vi "XY Graph Shift Plot Arrays.vi"(6 "Rotate":bool, 8 "Error In":errorcluster, 9 "Shift [index value] (0)":dbl, 10 "Y Array":dbl[](array[numeric]), 11 "X Array":dbl[](array[numeric])) -> (0 "Error Out":errorcluster, 2 "Y Array (shifted)":dbl[](array[numeric]), 3 "X Array (out)":dbl[](array[numeric]))   [LabVIEW 2021, in "XY Graph Add-Ons.lvlib"]
uses:
  XY Graph Add-Ons.lvlib
  9bdb4e87-38b8-4919-ab0a-2a6fc2bcb965.vi
  <vilib>/Utility/error.llb/Error Cluster From Error Code.vi
  <vilib>/ErrorRing/Error Ring.xnode
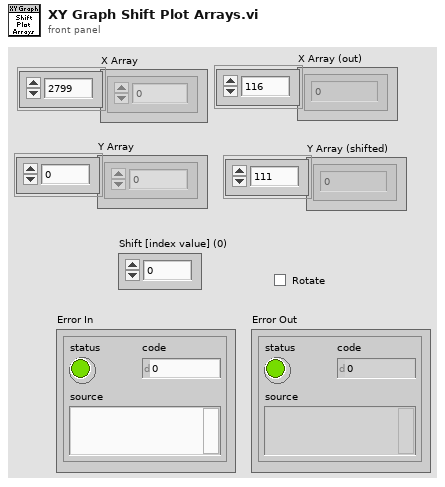
[diagram p1: front panel]
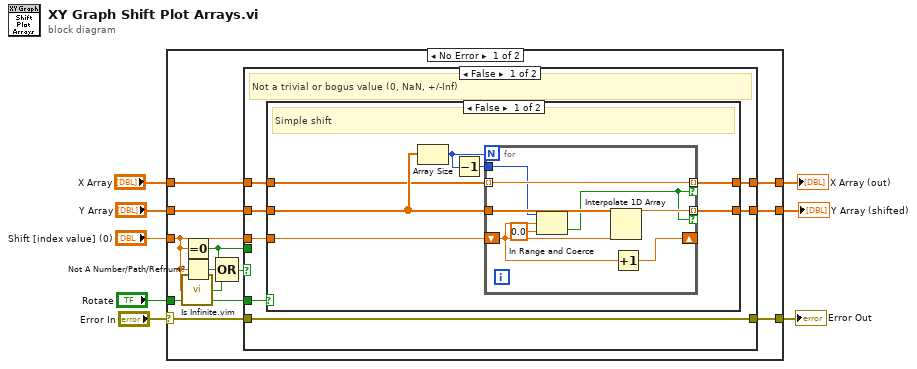
[diagram p0: block diagram]
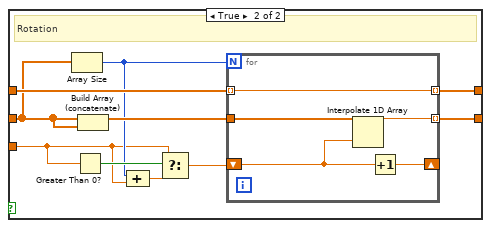
[diagram p2: hidden frame]
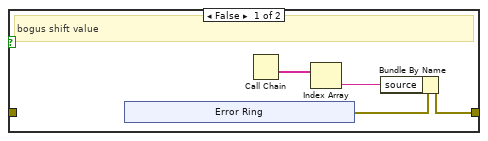
[diagram p4: hidden frame]
diagram:
  n1 = case shown="No Error" "Error In" {
    selector: "Error In" -> [w10 w72]
    tunnel: "Y Array" -> [w20 w74]
    tunnel: [w19 w74] -> w7
    tunnel: "Shift [index value] (0)" -> [w13 _]
    tunnel: "X Array" -> [w16 w73]
    tunnel: [w15 w73] -> w4
    tunnel: "Rotate" -> [w14 _]
    tunnel: [w9 w72] -> w1
    frame No Error {
      n2 = call "Is Infinite.vim"("Value"=w13) -> ("Is Infinite?"=w12:bool)
      n3 = Equal To 0?(x=w13) -> (x = 0?=w11:bool)
      n4 = Not A Number/Path/Refnum?(number/path/refnum=w13) -> (NaN/Path/Refnum?=w17:bool)
      n5 = Compound Arithmetic op=OR(w11, w17, w12) -> (w18:bool)
      n6 = case shown="False" w18 {
        tunnel: w20 -> [w27 w62]
        tunnel: [w26 w62] -> w19
        tunnel: w13 -> [w25 _]
        tunnel: w16 -> [w24 w61]
        tunnel: [w23 w61] -> w15
        tunnel: w14 -> [w22 _]
        tunnel: w11 -> [_ w60]
        tunnel: w10 -> [w21 w59]
        tunnel: [w21 w58] -> w9
        frame False {
          # "Not a trivial or bogus value (0, NaN, +/-Inf)"
          n7 = case shown="False" w22 {
            tunnel: w27 -> [w34 w49]
            tunnel: [w33 w52] -> w26
            tunnel: w25 -> [w32 w43]
            tunnel: w24 -> [w31 w51]
            tunnel: [w30 w50] -> w23
            frame False {
              # "Simple shift"
              n8 = Array Size(array=w34) -> (size(s)=w29:i32)
              n9 = Decrement(x=w29) -> (x-1=w28:i32)
              n10 = for {
                N: w29 -> [_]
                tunnel: w34 -> [w42]
                shift-right: [w40] -> _
                shift-left: w32 -> [w38]
                tunnel: [w41] -> w33 mode=indexing if=w35
                tunnel: w31 -> [w39] mode=indexing
                tunnel: [w39] -> w30 mode=indexing if=w35
                tunnel: w28 -> [w36]
                n11 = In Range and Coerce(upper limit=w36, x=w38, lower limit=0.0) -> (In Range?=w35:bool)  [unwired: 1 out]
                n12 = Interpolate 1D Array(1:w38, 2:w42) -> (0:w41:dbl)
                n13 = Increment(x=w38) -> (x+1=w40:dbl)
              }
            }
            frame True {
              # "Rotation"
              n14 = Array Size(array=w49) -> (size(s)=w46:i32)
              n15 = Greater Than 0?(x=w43) -> (x > 0?=w47:bool)
              n16 = Build Array (concatenate)(w49, w49) -> (w48:dbl[])
              n17 = Compound Arithmetic op=ADD(w46, w43) -> (w44:dbl)
              n18 = Select(t=w43, s=w47, f=w44) -> (s? t:f=w45:dbl)
              n19 = for {
                N: w46 -> [_]
                tunnel: w48 -> [w57]
                shift-right: [w55] -> _
                shift-left: w45 -> [w53]
                tunnel: [w56] -> w52 mode=indexing
                tunnel: w51 -> [w54] mode=indexing
                tunnel: [w54] -> w50 mode=indexing
                n20 = Interpolate 1D Array(1:w53, 2:w57) -> (0:w56:dbl)
                n21 = Increment(x=w53) -> (x+1=w55:dbl)
              }
            }
          }
        }
        frame True {
          n22 = case shown="True" w60 {
            tunnel: w59 -> [_ w71]
            tunnel: [w65 w71] -> w58
            frame False {
              # "bogus shift value"
              n23 = xnode "Error Ring"() -> ("error out"=w66:errorcluster)
              n24 = Call Chain() -> (call chain=w64:string[])
              n25 = Index Array(array=w64) -> (element=w63:string)  [unwired: 1 in]
              n26 = Bundle By Name(cluster=w66, "source"=w63) -> (w65:errorcluster)
            }
            frame True {
              # "no shift"
            }
          }
        }
      }
    }
    frame Error {
    }
  }
  "Y Array (shifted)" <- w7
  "Error Out" <- w1
  "X Array (out)" <- w4
